vi "PicoScope3000aExampleBlockMSO.vi"() -> ()   [LabVIEW 2010]
uses:
  shared/PicoBuffers.ctl
  <vilib>/Waveform/DWDTOps.llb/DWDT Analog to Digital.vi
  PicoScope3000aLib/PicoScope3000aAnalogChannelSettings.ctl
  PicoScope3000aLib/PicoScope3000aDigitalChannelSettings.ctl
  shared/Buffer and Transfer Settings.ctl
  shared/Acquisition Settings.ctl
panel:
  in  "Write to TDMS":bool
  in  "roundFaster":bool=TRUE
  in  "timeIntervalRequested":dbl min=0.0 format="%#6_6p"
  out "Pico 3000a Units":string
  in  "Trigger Settings":T1={"Trigger Enabled"=FALSE, "Trigger Source"=enum."Channel A", "Trigger Threshold (volts)"=0.0, "Trigger Direction"=2, "Trigger Delay (samples)"=0, "Auto Trigger Time (ms)"=1000} {"Trigger Direction" items=["Above", "Below", "Rising", "Falling", "Rising or Falling"]}
  in  "Channel A Settings":T2={"Enabled"=TRUE, "Coupling"=1, "Range"=6, "Analogue Offset"=0.0, "Bandwidth Limit"=0} {"Bandwidth Limit" items=["Full", "20MHz"]; "Range" items=["10 mV", "20 mV", "50 mV", "100 mV", "200 mV", "500 mV", "1 V", "2 V", "5 V", "10 V", "20 V", "50 V ", "100 V"]; "Coupling" items=["AC", "DC"]}
  in  "Port 0 Settings":T3={"Enabled"=FALSE, "Logic Level"=9830} {"Logic Level" items=["1.5V TTL"=9830, "2.5V CMOS"=16383]}
  out "overflow":i16 format="%010b"
  in  "Apply Settings":bool
  out "USB 3.0 device on non-USB 3.0 Port":bool=TRUE
  out "USB Powered":bool=TRUE
  out "Device Info":T4={"Driver Version"="2.1.104.3324", "USB Version"="2.0", "Hardware"="1", "Variant"="5244A", "Batch and Serial"="CQ178/007", "Cal Date"="11Jun13", "Kernel Version"="1.0", "Digital HW Version"="1", "Analogue HW Version"="1", "MSO"=FALSE, "Number of channels"=2}
  out "error out":errorcluster
  in  "Data file":path=path "PicoScope3000aExampleBlock Data"
  in  "Buffer and Transfer Settings":T5={"startIndex"=0, "Samples"=5000000, "Down Sample Ratio"=1, "Down-Sample Mode"=0} {"Down-Sample Mode" items=["RAW none"=2147483648, "None"=0, "Aggregate"=1, "Decimate"=2, "Average"=4]; "Down Sample Ratio" step=1; "Samples" format="%_6p"}
  in  "Acquisition Settings":T6={"preTriggerSamples"=0, "postTriggerSamples"=5000000, "timebase"=0} {"postTriggerSamples" format="%_6p"; "preTriggerSamples" format="%_6p"}
  out "Properties Panel":T7={"Sample Frequency"=41666668.0, "Sample Rate"=2.4000000209412065e-08, "Max Samples Available"=26843008, "Number of Samples"=0, "Total Capture Time (sec) "=0.0, "Max Total Capture Time Available (sec)"=0.6442322134971619} {"Max Total Capture Time Available (sec)" format="%.3p"; "Sample Frequency" format="%.6p"; "Sample Rate" format="%.3p"; "Max Samples Available" format="%_6p"; "Total Capture Time (sec)" format="%.3p"}
  out "Port 0":digitalwaveform(graph)={"t0"=timestamp(0 s since 1904-01-01), "dt"=8e-09, "Y"={"transitions"=[], "data"=[]}}
  in  "stop":bool
  out "Analog Channels":cluster{i32, sgl, "Data":dbl[]}[](graph)
  in  "Serial Number":string
  in  "Use Serial Number":bool
  in  "error in (no error)":errorcluster
  # "Bit 0 = ChA"
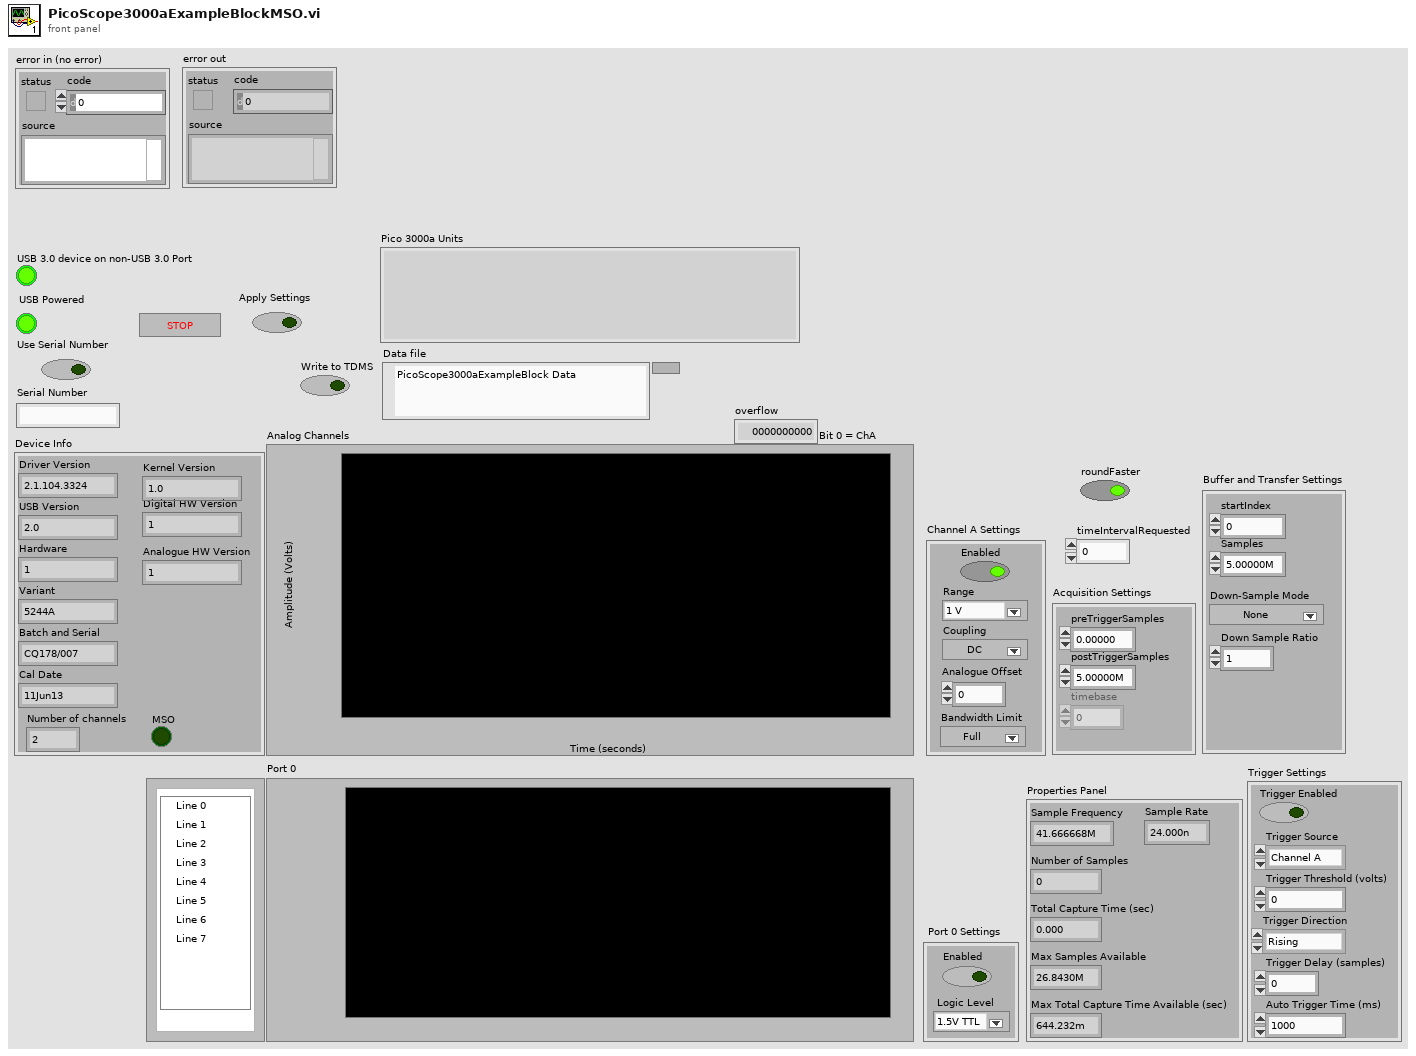
[diagram p1: front panel]
types:
  T1 = cluster{"Trigger Enabled":bool, "Trigger Source":enum32{"Channel A", "Channel B", "Channel C", "Channel D", "Ext."}, "Trigger Threshold (volts)":dbl, "Trigger Direction":u32, "Trigger Delay (samples)":u32, "Auto Trigger Time (ms)":i16}
  T2 = typedef "PicoScope3000aAnalogChannelSettings.ctl" = cluster{"Enabled":bool, "Coupling":u32, "Range":u32, "Analogue Offset":sgl, "Bandwidth Limit":u32}
  T3 = typedef "PicoScope3000aDigitalChannelSettings.ctl" = cluster{"Enabled":bool, "Logic Level":i16}
  T4 = cluster{"Driver Version":string, "USB Version":string, "Hardware":string, "Variant":string, "Batch and Serial":string, "Cal Date":string, "Kernel Version":string, "Digital HW Version":string, "Analogue HW Version":string, "MSO":bool, "Number of channels":i16}
  T5 = typedef "Buffer and Transfer Settings.ctl" = cluster{"startIndex":u64, "Samples":u64, "Down Sample Ratio":u64, "Down-Sample Mode":u32}
  T6 = typedef "Acquisition Settings.ctl" = cluster{"preTriggerSamples":u64, "postTriggerSamples":u64, "timebase":u32}
  T7 = cluster{"Sample Frequency":dbl, "Sample Rate":dbl, "Max Samples Available":u64, "Number of Samples":u64, "Total Capture Time (sec) ":dbl, "Max Total Capture Time Available (sec)":dbl}
  T8 = typedef "PicoBuffers.ctl" = cluster{"Max Buffer Pointers":u64[][][], "Min Buffer Pointers":u64[][][], "StreamingDataInfo":cluster{"Channel":u32, "Down-Sample Mode":u32, "PICO_DATA_TYPE":enum32{"PICO_INT8_T", "PICO_INT16_T", "PICO_INT32_T", "PICO_UINT32_T", "PICO_INT64_T", ""}, "Samples":i32, "bufferIndex":u64, "startIndex":i32, "overflow":i16}[][]}
  T9 = enum16{"open", "open or create", "create or replace", "create", "open (read-only)"}
  T10 = cluster{"Sample Frequency":sgl, "Sample Rate":sgl, "Max Samples Available":i32, "Number of Samples":u32, "Total Capture Time (sec) ":sgl, "Max Total Capture Time Available (sec)":sgl}
  T11 = cluster{"Channel A Buffer":i16[], "Channel B Buffer":i16[], "Channel C Buffer":i16[], "Channel D Buffer":i16[], "Channel E Buffer":i16[], "Channel F Buffer":i16[], "Channel G Buffer":i16[], "Channel H Buffer":i16[], "Port 0 Buffer":i16[], "Port 1 Buffer":i16[]}[]
  T12 = cluster{"Channel A Buffer":i16[], "Channel B Buffer":i16[], "Channel C Buffer":i16[], "Channel D Buffer":i16[], "Channel E Buffer":i16[], "Channel F Buffer":i16[], "Channel G Buffer":i16[], "Channel H Buffer":i16[], "Port 0 Buffer":i16[], "Port 1 Buffer":i16[]}
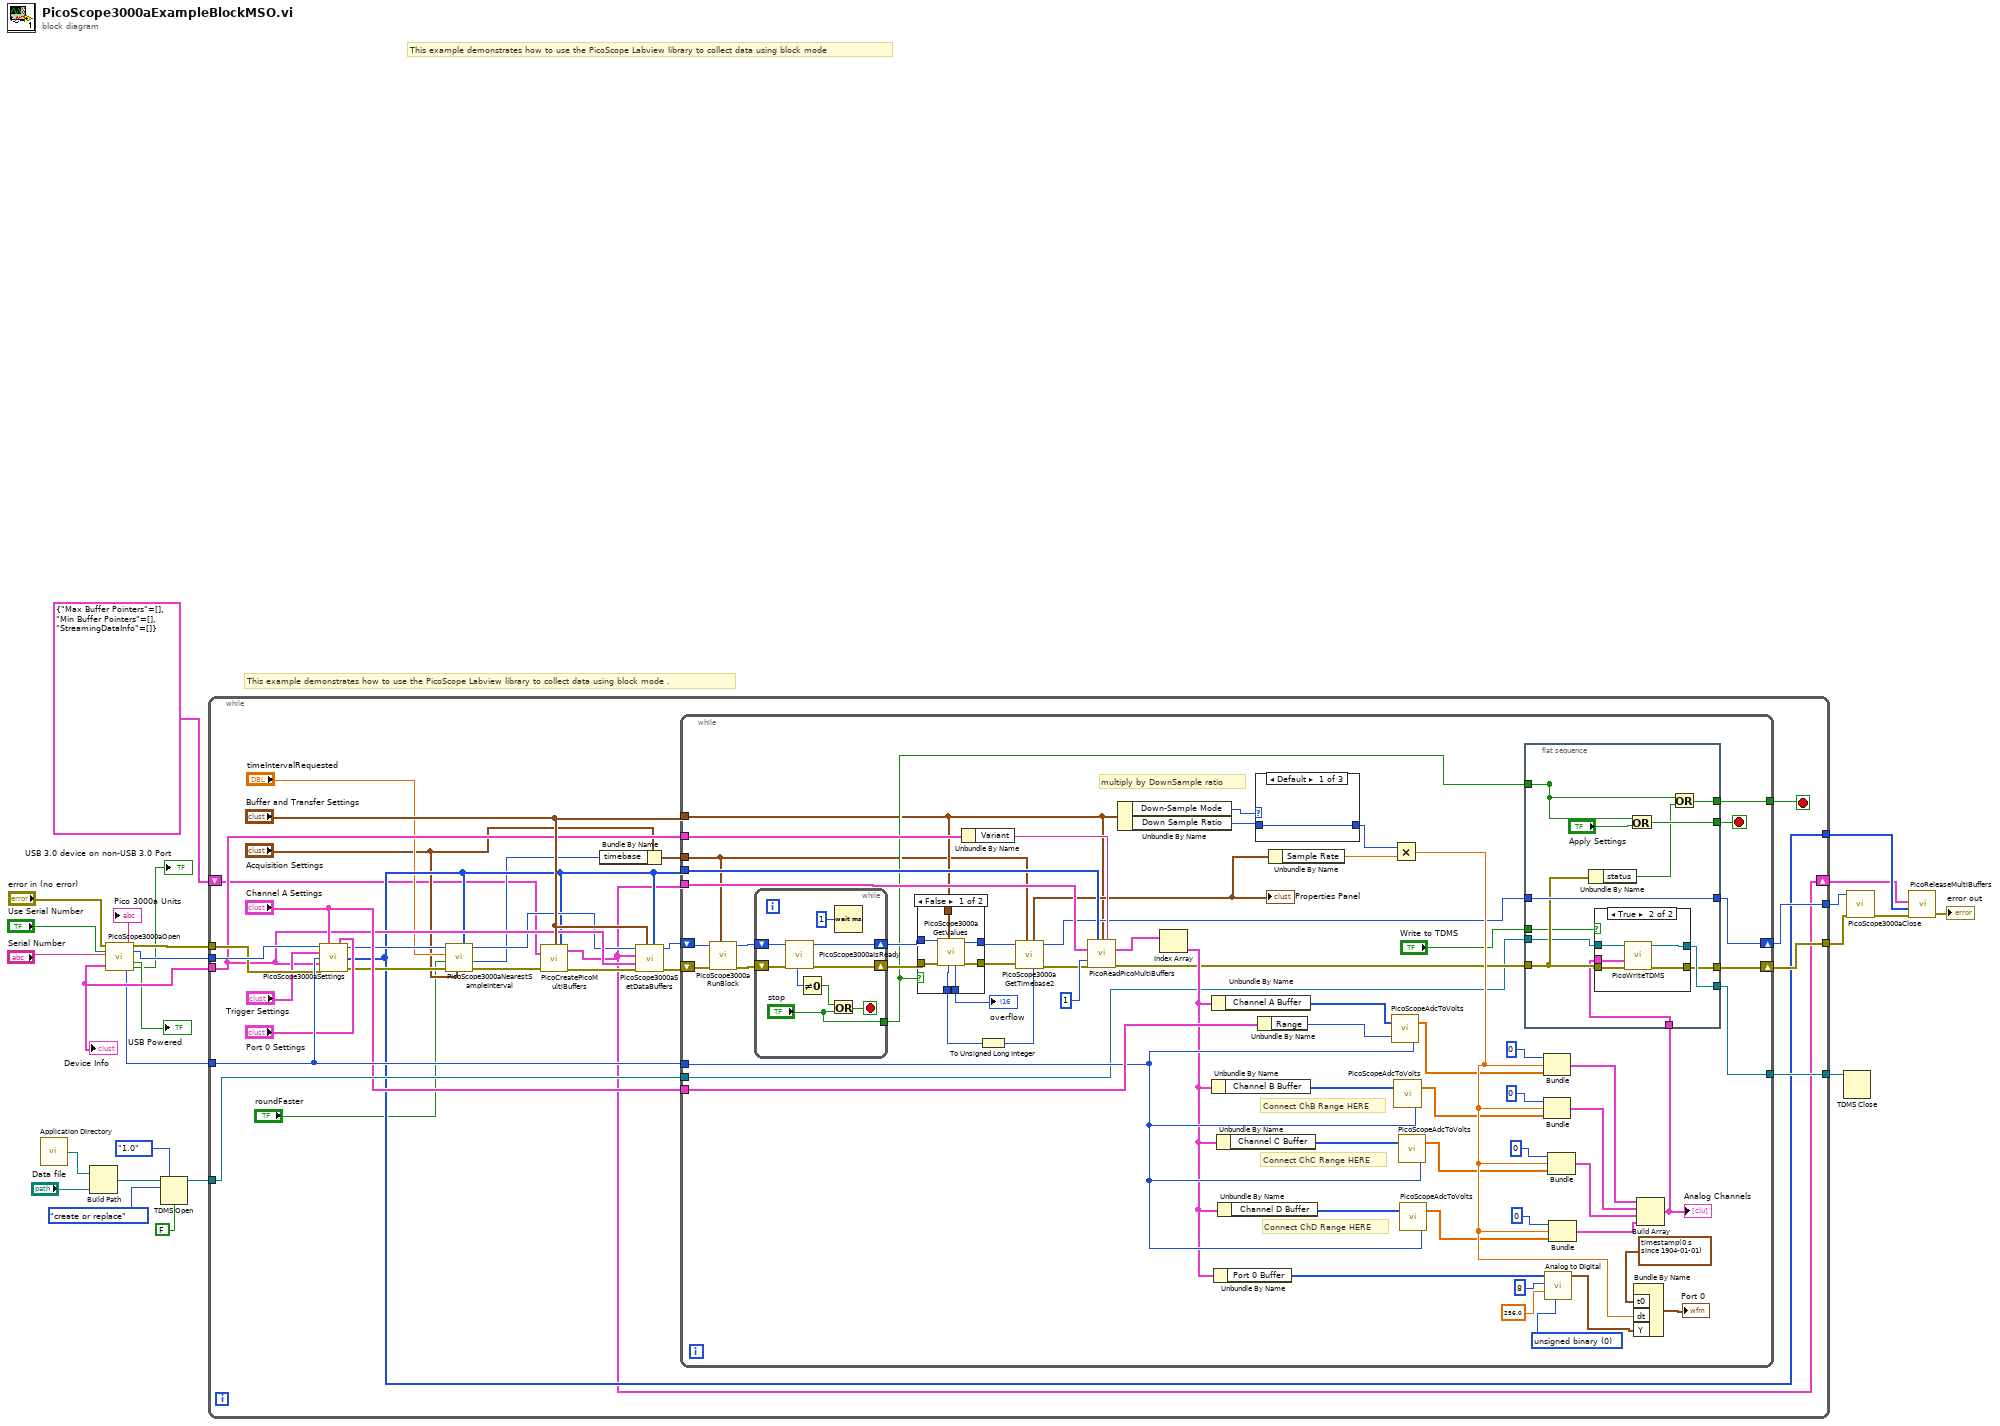
[diagram p0: block diagram]
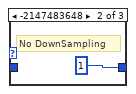
[diagram p4: hidden frame]
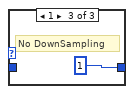
[diagram p5: hidden frame]
diagram:
  # "This example demonstrates how to use the PicoScope Labview library to collect data using block mode ."
  # "This example demonstrates how to use the PicoScope Labview library to collect data using block mode"
  n1 = call <vilib>:"Application Directory.vi"() -> ("Application Directory"=w18:path)
  n2 = Build Path(base path=w18, name or relative path="Data file") -> (appended path=w19:path)
  n3 = call "PicoScope3000aOpen.vi"("error in (no error)"="error in (no error)", "Serial Number"="Serial Number", "Use Serial number"="Use Serial Number") -> ("Pico 3000a Units"=→"Pico 3000a Units":string, "error out"=w9:errorcluster, "handle"=w25:i16, "USB Powered"=→"USB Powered":bool, "Device Info"=w11:T4, "Max ADC value"=w8:i16, "USB 3.0 device on non-USB 3.0 Port"=→"USB 3.0 device on non-USB 3.0 Port":bool)  [unwired: 6 in]
  "Device Info" <- w11
  n4 = TDMS Open(6:FALSE ("disable buffering? (T)"), 7:enum16{"1.0", "2.0"}."1.0" ("file format version (2.0)"), 10:T9."create or replace" ("operation (0:open)"), 11:w19) -> (3:w16:refnum<k34>)  [unwired: 2 in, 1 out]
  n5 = while {
    tunnel: w25 -> [w42]
    tunnel: w8 -> [w44]
    tunnel: [w33] -> w24
    tunnel: [w50] -> w17
    tunnel: w16 -> [w52]
    tunnel: w11 -> [w38]
    tunnel: w9 -> [w41]
    tunnel: [w51] -> w5
    tunnel: [w48] -> w3
    shift-right: [w26] -> w1
    shift-left: T8 {"Max Buffer Pointers"=[], "Min Buffer Pointers"=[], "StreamingDataInfo"=[]} ("Data Pointers") -> [w27]
    stop <- w49 stop-if-true
    n6 = call "PicoScope3000aSettings.vi"("handle in"=w42, "Channel A Settings"="Channel A Settings", "Port 0 Settings"="Port 0 Settings", "Trigger Settings"="Trigger Settings", "Max_adc"=w44, "Device Info"=w38, "error in"=w41) -> ("handle out"=w34:i16, "Enabled Array"=w33:i16[], "error out"=w37:errorcluster)  [unwired: 6 in]
    n7 = call "PicoScope3000aNearestSampleInterval.vi"("Enabled array"=w33, "Acquisition Settings"="Acquisition Settings", "error in (no error)"=w37, "roundFaster"="roundFaster", "timeIntervalRequested"="timeIntervalRequested", "handle in"=w34) -> ("error out"=w36:errorcluster, "timebase"=w31:u32, "handle out"=w35:i16)  [unwired: 2 in, 1 out]
    n8 = call "PicoCreatePicoMultiBuffers.vi"("Buffer and Transfer Settings"="Buffer and Transfer Settings", "enabled array"=w33, "Data Pointers In"=w27, "error in (no error)"=w36) -> ("Data Pointers"=w26:T8, "error out"=w53:errorcluster)  [unwired: 10 in]
    n9 = Bundle By Name(cluster="Acquisition Settings", "timebase"=w31) -> (w32:T6)
    n10 = call "PicoScope3000aSetDataBuffers.vi"("enabled array"=w33, "Buffer and Transfer Settings"="Buffer and Transfer Settings", "error in (no error)"=w53, "Device Info"=w38, "Data Pointers In"=w26, "handle in"=w35) -> ("error out"=w47:errorcluster, "handle out"=w46:i16)  [unwired: 4 in]
    n11 = while {
      tunnel: w26 -> [w117]
      tunnel: "Buffer and Transfer Settings" -> [w58]
      tunnel: w33 -> [w109]
      tunnel: "Channel A Settings" -> [w108]
      tunnel: w32 -> [w57]
      tunnel: w44 -> [w107]
      tunnel: w38 -> [w104]
      tunnel: [w74] -> w49
      shift-right: [w77] -> w51
      shift-left: w47 -> [w68]
      shift-right: [w72] -> w48
      shift-left: w46 -> [w69]
      tunnel: w52 -> [w55]
      tunnel: [w76] -> w50
      stop <- w73 stop-if-true
      w94 = u16 0 items=["unsigned binary", "offset binary", "2's complement"] ("data format (offset binary)")
      # "Connect ChB Range HERE"
      # "Connect ChD Range HERE"
      # "Connect ChC Range HERE"
      # "multiply by DownSample ratio"
      n12 = call "PicoScope3000aRunBlock.vi"("Acquisition Settings"=w57, "error in (no error)"=w68, "handle in"=w69) -> ("error out"=w111:errorcluster, "handle out"=w110:i16)  [unwired: 5 in, 2 out]
      n13 = while {
        shift-right: [w153] -> w70
        shift-left: w111 -> [w154]
        shift-right: [w152] -> w71
        shift-left: w110 -> [w151]
        tunnel: ["stop"] -> w67
        stop <- w148 stop-if-true
        n14 = call "PicoScope3000aIsReady.vi"("error in (no error)"=w154, "handle in"=w151) -> ("error out"=w153:errorcluster, "handle out"=w152:i16, "ready"=w150:i16)  [unwired: 7 in]
        n15 = Not Equal To 0?(x=w150) -> (x != 0?=w149:bool)
        n16 = Or(x=w149, y="stop") -> (x .or. y?=w148:bool)
        n17 = Wait (ms)(milliseconds to wait=u32 1) -> ()  [unwired: 1 out]
      }
      n18 = case shown="False" w67 {
        tunnel: w70 -> [w124 w125]
        tunnel: w71 -> [w123 w126]
        tunnel: [w122 w126] -> w63
        tunnel: [w121 w125] -> w64
        tunnel: w58 -> [w120 _]
        tunnel: [w119 _] -> w66
        tunnel: [w118 _] -> w60
        frame False {
          n19 = call "PicoScope3000aGetValues.vi"("Buffer and Transfer Settings"=w120, "error in (no error)"=w124, "handle in"=w123) -> ("error out"=w121:errorcluster, "handle out"=w122:i16, "overflow"=w119:i16, "noOfSamples"=w118:u64)  [unwired: 5 in]
        }
        frame True {
        }
      }
      "overflow" <- w66
      n20 = Unbundle By Name(w104) -> ("Variant"=w105:string)
      n21 = To Unsigned Long Integer(number=w60) -> (unsigned 32bit integer=w59:u32)
      n22 = call "PicoScope3000aGetTimebase2.vi"("Number of Samples"=w59, "Acquisition Settings"=w57, "error in (no error)"=w64, "handle in"=w63) -> ("error out"=w62:errorcluster, "handle out"=w61:i16, "Properties Panel"=w65:T10)  [unwired: 5 in]
      "Properties Panel" <- w65
      n23 = call "PicoReadPicoMultiBuffers.vi"("enabled array"=w109, "Buffer and Transfer Settings"=w58, "Variant"=w105, "Data Pointers"=w117, "No of Buffers"=1, "error in (no error)"=w62) -> ("MultiBuffers (Max or non-aggregated)"=w116:T11, "error out"=w75:errorcluster)  [unwired: 7 in, 1 out]
      n24 = Unbundle By Name(w58) -> ("Down-Sample Mode"=w114:u32, "Down Sample Ratio"=w115:u64)
      n25 = Index Array(array=w116) -> (element=w78:T12)  [unwired: 1 in]
      n26 = Unbundle By Name(w78) -> ("Channel A Buffer"=w87:i16[])
      n27 = Unbundle By Name(w78) -> ("Channel B Buffer"=w99:i16[])
      n28 = Unbundle By Name(w78) -> ("Port 0 Buffer"=w92:i16[])
      n29 = Unbundle By Name(w78) -> ("Channel C Buffer"=w85:i16[])
      n30 = Unbundle By Name(w78) -> ("Channel D Buffer"=w81:i16[])
      n31 = case shown="Default" w114 {
        tunnel: [w155 u64 1 ("Down Sample Ratio") u64 1 ("Down Sample Ratio")] -> w112
        tunnel: w115 -> [w155 _ _]
        frame Default {
        }
        frame -2147483648 {
          # "No DownSampling"
        }
        frame 1 {
          # "No DownSampling"
        }
      }
      n32 = Unbundle By Name(w108) -> ("Range"=w101:u32)
      n33 = Unbundle By Name(w65) -> ("Sample Rate"=w106:sgl)
      n34 = call "PicoScopeAdcToVolts.vi"("Max_adc"=w107, "Range Index"=w101, "Data"=w87) -> ("Data"=w88:dbl[])
      n35 = Multiply(x=w112, y=w106) -> (x*y=w113:sgl)
      n36 = call "PicoScopeAdcToVolts.vi"("Max_adc"=w107, "Data"=w99) -> ("Data"=w98:dbl[])  [unwired: 1 in]
      n37 = call "PicoScopeAdcToVolts.vi"("Max_adc"=w107, "Data"=w85) -> ("Data"=w84:dbl[])  [unwired: 1 in]
      n38 = call "PicoScopeAdcToVolts.vi"("Max_adc"=w107, "Data"=w81) -> ("Data"=w80:dbl[])  [unwired: 1 in]
      n39 = flat-sequence {
        tunnel: [w138] -> w73
        tunnel: [w133] -> _
        tunnel: [w135] -> w74
        tunnel: w61 -> [w134]
        tunnel: [w134] -> w72
        tunnel: w75 -> [w130]
        tunnel: [w131] -> w77
        tunnel: [w132] -> w76
        tunnel: w67 -> [w133]
        tunnel: w56 -> [w129]
        tunnel: w55 -> [w128]
        tunnel: "Write to TDMS" -> [w127]
        frame #0 {
          n40 = Unbundle By Name(w130) -> ("status"=w136:bool)
          n41 = case shown="True" w127 {
            tunnel: w129 -> [_ w145]
            tunnel: w128 -> [w139 w144]
            tunnel: w130 -> [w140 w143]
            tunnel: [w140 w142] -> w131
            tunnel: [w139 w141] -> w132
            frame False {
            }
            frame True {
              n42 = call "PicoWriteTDMS.vi"("error in (no error)"=w143, "Analog Channels"=w145, "Refnum in"=w144) -> ("error out"=w142:errorcluster, "Refnum out"=w141:refnum<k34>)  [unwired: 7 in]
            }
          }
          n43 = Or(x=w133, y="Apply Settings") -> (x .or. y?=w138:bool)
          n44 = Or(x=w133, y=w136) -> (x .or. y?=w135:bool)
        }
      }
      n45 = Bundle(0, w113, "Data"=w88) -> (w97:cluster{i32, sgl, "Data":dbl[]})  [unwired: 1 in]
      n46 = Bundle(0, w113, "Data"=w98) -> (w96:cluster{i32, sgl, "Data":dbl[]})  [unwired: 1 in]
      n47 = call-poly <vilib>:"Analog to Digital.vi"("data format (offset binary)"=w94, "full-scale range (pk-pk)"=256.0, "resolution (16 bit)"=8, "analog waveform"=w92) -> ("digital waveform"=w89:digitalwaveform)  [unwired: 4 in, 3 out]
      n48 = Bundle(0, w113, "Data"=w84) -> (w83:cluster{i32, sgl, "Data":dbl[]})  [unwired: 1 in]
      n49 = Bundle(0, w113, "Data"=w80) -> (w79:cluster{i32, sgl, "Data":dbl[]})  [unwired: 1 in]
      n50 = Bundle By Name("t0"=timestamp(0 s since 1904-01-01), "dt"=w113, "Y"=w89) -> (→"Port 0":digitalwaveform)  [unwired: 1 in]
      n51 = Build Array(w97, w96, w83, w79) -> (w56:cluster{i32, sgl, "Data":dbl[]}[])
      "Analog Channels" <- w56
    }
  }
  n52 = TDMS Close(11:w17) -> ()  [unwired: 1 in, 2 out]
  n53 = call "PicoScope3000aClose.vi"("error in (no error)"=w5, "handle in"=w3) -> ("error out"=w4:errorcluster)  [unwired: 8 in, 1 out]
  n54 = call "PicoReleaseMultiBuffers.vi"("error in (no error)"=w4, "Enabled array"=w24, "Data Pointers"=w1) -> ("error out"=→"error out":errorcluster)  [unwired: 7 in, 1 out]
